vi "PowerSupplyRemoteCommandsToChangeTheLED_Intensity.vi"() -> ()   [LabVIEW 2022 SP3]
panel:
  in  "error in (no error)":errorcluster
  in  "VISA resource name":refnum<visa-resource-name>
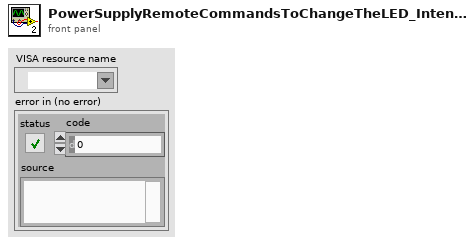
[diagram p1: front panel]
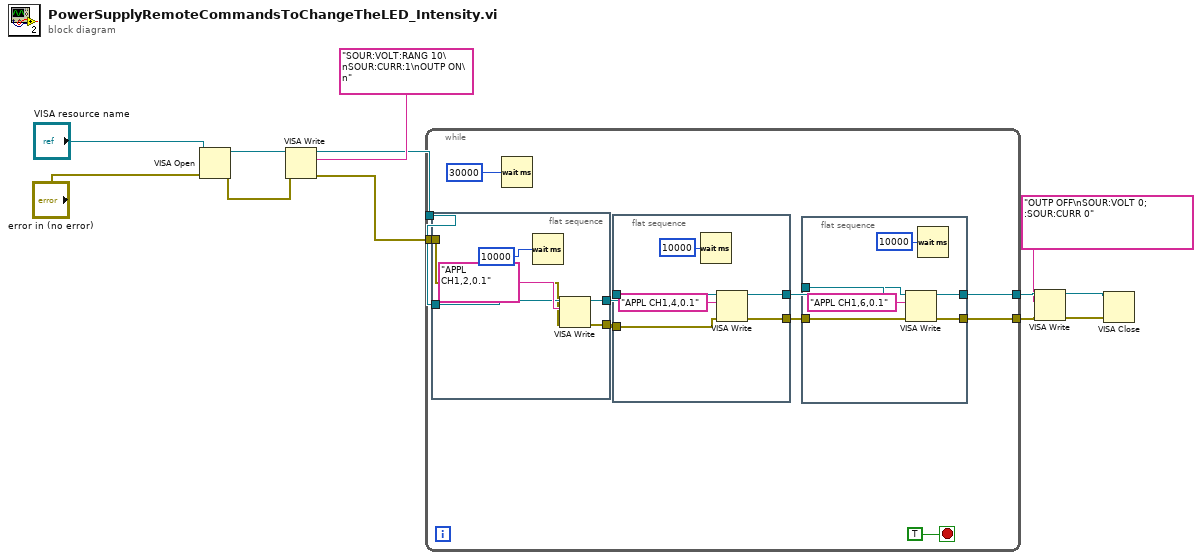
[diagram p0: block diagram]
diagram:
  n1 = VISA Open(error in (no error)="error in (no error)", VISA resource name="VISA resource name") -> (VISA resource name=w12:refnum<visa-resource-name>, error out=w8:errorcluster)  [unwired: 3 in]
  n2 = VISA Write(VISA resource name=w12, write buffer="SOUR:VOLT:RANG 10\nSOUR:CURR:1\nOUTP ON\n", error in (no error)=w8) -> (VISA resource name out=w7:refnum<visa-resource-name>, error out=w6:errorcluster)  [unwired: 1 out]
  n3 = while {
    tunnel: w7 -> [w21]
    tunnel: w6 -> [w20]
    tunnel: [w15] -> w5
    tunnel: [w14] -> w4
    stop <- TRUE stop-if-true
    n4 = flat-sequence {
      tunnel: w21 -> [w26]
      tunnel: w20 -> [w25]
      tunnel: [w24] -> w19
      tunnel: [w23] -> w18
      frame #0 {
        n5 = Wait (ms)(milliseconds to wait=u32 10000) -> ()  [unwired: 1 out]
        n6 = VISA Write(VISA resource name=w26, write buffer="APPL CH1,2,0.1", error in (no error)=w25) -> (VISA resource name out=w24:refnum<visa-resource-name>, error out=w23:errorcluster)  [unwired: 1 out]
      }
    }
    n7 = Wait (ms)(milliseconds to wait=u32 30000) -> ()  [unwired: 1 out]
    n8 = flat-sequence {
      tunnel: w19 -> [w39]
      tunnel: w18 -> [w38]
      tunnel: [w36] -> w17
      tunnel: [w35] -> w16
      frame #0 {
        n9 = Wait (ms)(milliseconds to wait=u32 10000) -> ()  [unwired: 1 out]
        n10 = VISA Write(VISA resource name=w39, write buffer="APPL CH1,4,0.1", error in (no error)=w38) -> (VISA resource name out=w36:refnum<visa-resource-name>, error out=w35:errorcluster)  [unwired: 1 out]
      }
    }
    n11 = flat-sequence {
      tunnel: w17 -> [w33]
      tunnel: w16 -> [w32]
      tunnel: [w30] -> w15
      tunnel: [w29] -> w14
      frame #0 {
        n12 = VISA Write(VISA resource name=w33, write buffer="APPL CH1,6,0.1", error in (no error)=w32) -> (VISA resource name out=w30:refnum<visa-resource-name>, error out=w29:errorcluster)  [unwired: 1 out]
        n13 = Wait (ms)(milliseconds to wait=u32 10000) -> ()  [unwired: 1 out]
      }
    }
  }
  n14 = VISA Write(VISA resource name=w5, write buffer="OUTP OFF\nSOUR:VOLT 0; :SOUR:CURR 0", error in (no error)=w4) -> (VISA resource name out=w2:refnum<visa-resource-name>, error out=w1:errorcluster)  [unwired: 1 out]
  n15 = VISA Close(VISA resource name=w2, error in (no error)=w1) -> ()  [unwired: 1 out]
